vi "greatestOutlier.vi"(10 "line in":cluster{"X":dbl, "Y":dbl}[](array[cluster])) -> (1 "max index":i32, 2 "max value":dbl)   [LabVIEW 2016]
uses:
  <vilib>/Analysis/NI_AALPro.lvlib
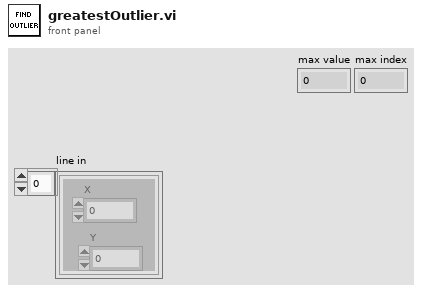
[diagram p1: front panel]
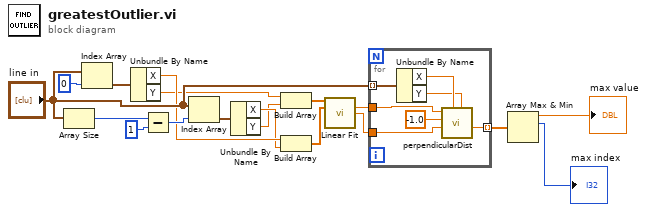
[diagram p0: block diagram]
diagram:
  n1 = Array Size(array="line in") -> (size(s)=w11:i32)
  n2 = Index Array(array="line in", index=0) -> (element=w8:cluster{"X":dbl, "Y":dbl})
  n3 = Unbundle By Name(w8) -> ("X"=w6:dbl, "Y"=w4:dbl)
  n4 = Subtract(x=w11, y=1) -> (x-y=w10:i32)
  n5 = Index Array(array="line in", index=w10) -> (element=w7:cluster{"X":dbl, "Y":dbl})
  n6 = Unbundle By Name(w7) -> ("X"=w5:dbl, "Y"=w3:dbl)
  n7 = Build Array(w4, w3) -> (w2:dbl[])
  n8 = Build Array(w6, w5) -> (w1:dbl[])
  n9 = call <vilib>:"Linear Fit.vi"("Y"=w2, "X"=w1) -> ("slope"=w18:dbl, "intercept"=w17:dbl)  [unwired: 9 in, 3 out]
  n10 = for {
    tunnel: "line in" -> [w25] mode=indexing
    tunnel: w18 -> [w22]
    tunnel: w17 -> [w21]
    tunnel: [w19] -> w16 mode=indexing
    n11 = Unbundle By Name(w25) -> ("X"=w24:dbl, "Y"=w23:dbl)
    n12 = call "perpendicularDist.vi"("Y2"=w23, "X1"=w24, "C"=w21, "B"=-1.0, "A"=w22) -> ("Distance"=w19:dbl)  [unwired: 6 in]
  }
  n13 = Array Max & Min(array=w16) -> (max value=→"max value":dbl, max index (indices)=→"max index":i32)  [unwired: 2 out]
